vi "Configure.vi"(8 "error in (no error)":errorcluster, 11 "GRMActor in":refnum<class "StepMotorController.lvclass">) -> (0 "error out":errorcluster, 3 "GRMActor out":refnum<class "StepMotorController.lvclass">)   [LabVIEW 2020, in "StepMotorController.lvlib" / "StepMotorController.lvclass"]
uses:
  StepMotorController.lvclass
  Model/Hardware Abstraction Layer/Component/GenericActor/GenericActor/GenericController.lvclass
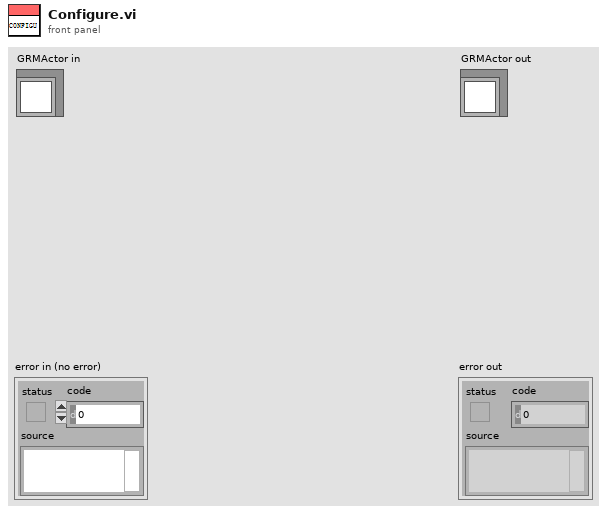
[diagram p1: front panel]
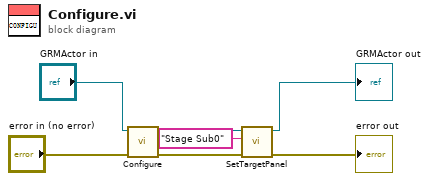
[diagram p0: block diagram]
diagram:
  n1 = call-parent "Configure.vi"("error in (no error)"="error in (no error)", "GRMActor in"="GRMActor in") -> ("error out"=w7:errorcluster, "GRMActor out"=w3:refnum<class "StepMotorController.lvclass">)  [unwired: 8 in]
  n2 = call-dynamic "SetTargetPanel.vi"("error in (no error)"=w7, "TargetPanel"="Stage Sub0", "GRMActor in"=w3) -> ("error out"=→"error out":errorcluster, "GRMActor out"=→"GRMActor out":refnum<class "StepMotorController.lvclass">)  [unwired: 7 in]
